vi "Word Edit Cell.vi"   [LabVIEW 2020, in "NI_ReportGenerationToolkit.lvlib"]
doc: "Edits the cell specified by the <B>row</B> and <B>column</B> elements of the <B>start</B> input. The data type you wire to the <B>value</B> input determines the polymorphic instance to use."
uses:
  <vilib>/addons/_office/NI_ReportGenerationToolkit.lvlib
  <vilib>/Utility/NIReport.llb/Word/NI_Word.lvclass
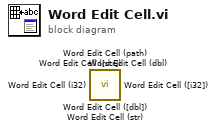
[diagram p0: block diagram]
diagram:
  n1 = call <vilib>:"Word Edit Cell ([dbl]).vi"() -> ()  [unwired: 14 in, 2 out]
  n2 = call <vilib>:"Word Edit Cell (dbl).vi"() -> ()  [unwired: 14 in, 2 out]
  n3 = call <vilib>:"Word Edit Cell (i32).vi"() -> ()  [unwired: 14 in, 2 out]
  n4 = call <vilib>:"Word Edit Cell ([i32]).vi"() -> ()  [unwired: 14 in, 2 out]
  n5 = call <vilib>:"Word Edit Cell (str).vi"() -> ()  [unwired: 14 in, 2 out]
  n6 = call <vilib>:"Word Edit Cell (path).vi"() -> ()  [unwired: 14 in, 2 out]
  n7 = call <vilib>:"Word Edit Cell ([str]).vi"() -> ()  [unwired: 14 in, 2 out]
